vi "IECMemory.LoadRamp.vi"(0 "i ref in":refnum<vi>, 1 "FirstStep":i32, 2 "SecondStep":i32, 3 "ms timeout (100)":i32=100, 5 "error in (no error)":errorcluster) -> (14 "i ref out":refnum<vi>, 17 "timed out":bool, 19 "error out":errorcluster)   [LabVIEW 2014, in "IECMemory.lvlib"]
uses:
  IECMemory.lvlib
  CSCore/CSSystem/CoreDefs/CoreDefs.error_type.ctl
  CSCore/CSSystem/CoreLib/CoreLib.lvlib
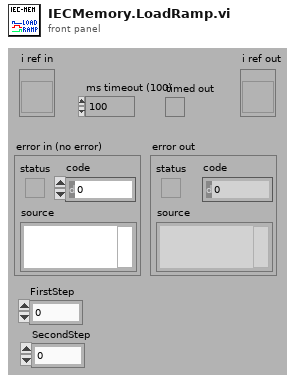
[diagram p1: front panel]
types:
  T1 = typedef "CoreDefs.error_type.ctl" = enum16{"no error", "can't load process", "can't unload process", "process does not exist", "can't install process", "can't remove process", "unknown function", "time out", "can't execute function", "duplicate queue name", "super not found", "caller queue invalid", "can't ping process", "unknown error", "VISA Error", "VISA timeout", "GPIB timeout", "GPIB error", "communication error", "data type mismatch", "can't read data from OPC server", "can't write data to OPC server", "OET error", "function not implemented", "process already exists", "invalid Shared Variable name", "error writing Shared Variable", "error reading Shared Variable", "invalid client name", "corrupt database", "unknown class", "call not authorized", "parameter out of range", "OET timeout: can't get data to modify", "invalid queue name", "requested operation incompatible with current state", "event undefined", "event disabled", "state undefined", "caller is not a friend", "EventBuilder: bad eventID", "EventBuilder: no DAQ devices", "a thread must not stop itself", "UNUSED ELEMENT4", "DiscArchiver: eventData incomplete", "DiscArchiver: eventData does not belong to run", "DiscArchiver: can't open file", "DiscArchiver: can't write to file", "DiscArchiver: available disc space low", "can't acquire semaphore", "error reading data from database", "notifier object is not existing", "can't register process", "can't unregister process", "illegal event type", "object disabled", "object already exists", "can't change state", "Instrument not found", "no connection to remote node", "invalid reference", "N/A", "UNUSED ELEMENT 1", "element not found", "illegal TCP/IP connection detected", "object does not exist", "invalid access ID", "unknown CS system", "invalid privilige", "unsupported data type", "unsupported server type", "IO server already exists", "Shared Variable already exists"}
  T2 = typedef "IECMemory.lvlib/IECMemory.i attribute.ctl" = cluster{"EndAddress":u32, "MemoryStatusBits":T3, "IEC Finished":bool, "Call Process":string, "Call Event":string}
  T3 = typedef "IECMemoryDriver.lvlib/Memory_Status.ctl" = bool[]
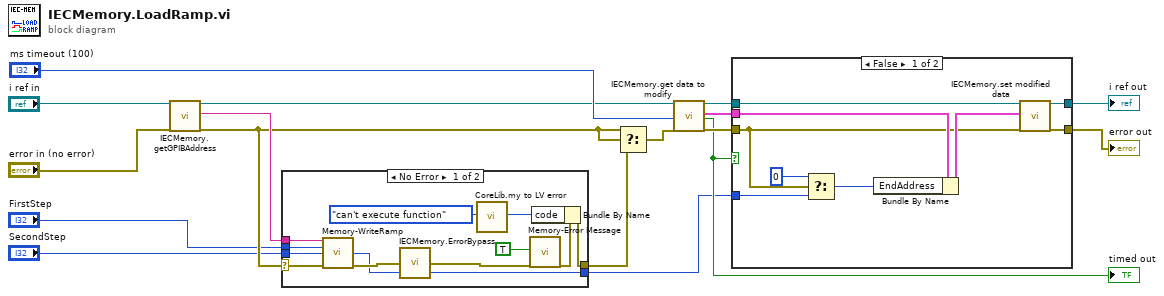
[diagram p0: block diagram]
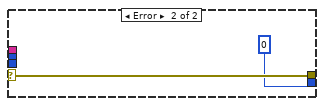
[diagram p2: hidden frame]
diagram:
  n1 = call "IECMemory.getGPIBAddress.vi"("i ref in"="i ref in", "error in (no error)"="error in (no error)") -> ("i ref out"=w11:refnum<vi>, "GPIBAddress"=w7:string, "error out"=w4:errorcluster)  [unwired: 14 in, 1 out]
  n2 = case shown="No Error" w4 {
    selector: w4 -> [w24 w31]
    tunnel: [w26 w31] -> w3
    tunnel: [w20 u32 0] -> w6
    tunnel: w7 -> [w22 _]
    tunnel: "FirstStep" -> [w19 _]
    tunnel: "SecondStep" -> [w21 _]
    frame No Error {
      n3 = call "Memory-WriteRamp.vi"("AddressStringIN"=w22, "FirstStep"=w19, "SecondStep"=w21, "error in (no error)"=w24) -> ("EndAddress"=w20:i16, "error out"=w23:errorcluster)  [unwired: 10 in]
      n4 = call "IECMemory.ErrorBypass.vi"("error in (no error)"=w23) -> ("error out"=w18:errorcluster)  [unwired: 14 in]
      n5 = call "CoreLib.my to LV error.vi"("ErrorTypes"=CoreDefs.error_type."can't execute function") -> ("LV error code"=w25:i32)  [unwired: 17 in, 1 out]
      n6 = call "Memory-Error Message.vi"("add message to source"=TRUE, "error in (no error)"=w18) -> ("error out"=w27:errorcluster)  [unwired: 14 in, 3 out]
      n7 = Bundle By Name(cluster=w27, "code"=w25) -> (w26:errorcluster)
    }
    frame Error {
    }
  }
  n8 = Select(t=w4, s=w4, f=w3) -> (s? t:f=w5:errorcluster)
  n9 = call "IECMemory.get data to modify.vi"("i ref in"=w11, "ms timeout (10000)"="ms timeout (100)", "error in (no error)"=w5) -> ("i ref out"=w15:refnum<vi>, "i attribute"=w13:T2, "timed out"=w10:bool, "error out"=w14:errorcluster)  [unwired: 13 in]
  "timed out" <- w10
  n10 = case shown="False" w10 {
    tunnel: w15 -> [w36 w42]
    tunnel: [w38 w42] -> w9
    tunnel: [w37 w41] -> w8
    tunnel: w14 -> [w34 w41]
    tunnel: w13 -> [w40 _]
    tunnel: w6 -> [w32 _]
    frame False {
      n11 = Select(t=u32 0, s=w34, f=w32) -> (s? t:f=w39:u32)
      n12 = Bundle By Name(cluster=w40, "EndAddress"=w39) -> (w35:T2)
      n13 = call "IECMemory.set modified data.vi"("i ref in"=w36, "i attribute"=w35, "error in (no error)"=w34) -> ("i ref out"=w38:refnum<vi>, "error out"=w37:errorcluster)  [unwired: 15 in]
    }
    frame True {
    }
  }
  "error out" <- w8
  "i ref out" <- w9
